vi "SetFrameRate.vi"(8 "error in (no error)":errorcluster, 10 "Frame Rate (hex code)":u8 caption="Frame Rate" format="%.0x", 11 "CameraDemo in":refnum<class "CameraDemo.lvclass">) -> (0 "error out":errorcluster, 3 "CameraDemo out":refnum<class "CameraDemo.lvclass">)   [LabVIEW 2020, in "CameraI2COUSB.lvlib" / "CameraDemo.lvclass"]
uses:
  CameraDemo.lvclass
  CameraDemo.lvclass/CameraDemo.ctl
  Private/TypeDef/RegisterName.ctl
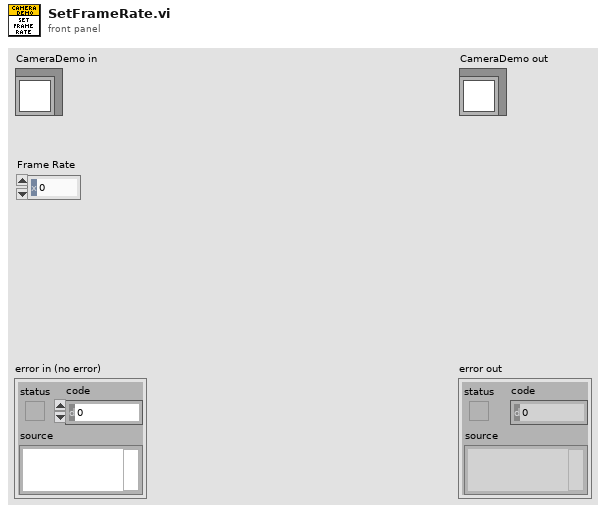
[diagram p1: front panel]
types:
  T1 = typedef "CameraI2COUSB.lvlib/CameraDemo.lvclass/RegisterName.ctl" = enum16{"Clock Rate", "Frame Rate", "Image Type", "Resolution", "Snap", "Start Streaming", "Stop Streaming"}
  T2 = typedef "CameraI2COUSB.lvlib/CameraDemo.lvclass/RegisterInfo.ctl" = cluster{"Address":u16, "Lenght":u32}
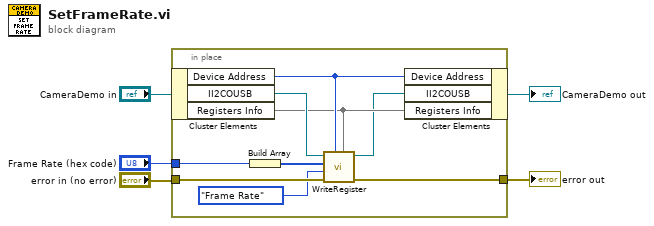
[diagram p0: block diagram]
diagram:
  n1 = in-place {
    in-place-border: "error in (no error)" -> [w14]
    in-place-border: "Frame Rate (hex code)" -> [w9]
    in-place-border: [w7] -> w1
    n2 = in-place-cluster #1("CameraDemo in") -> ("Device Address"=w13:u8, "II2COUSB"=w12:refnum<class "II2COUSB.lvclass">, "Registers Info"=w11:map{T1, T2})
    n3 = Build Array(w9) -> (w8:u8[])
    n4 = call "WriteRegister.vi"("Registers Info"=w11, "Device Address"=w13, "error in (no error)"=w14, "Register Name"=RegisterName."Frame Rate", "DATA"=w8, "II2COUSB"=w12) -> ("error out"=w7:errorcluster, "II2COUSB out"=w6:refnum<class "II2COUSB.lvclass">)  [unwired: 4 in]
    n5 = in-place-cluster #1("Device Address"=w13, "II2COUSB"=w6, "Registers Info"=w11) -> (→"CameraDemo out":refnum<class "CameraDemo.lvclass">)
  }
  "error out" <- w1
